vi "Mark Points Holder.vi"(2 "Actions":T1=enum."Read", 7 "(X, Y) Points":dbl[](array[numeric]), 13 "Zero Position (x, y)":dbl[](array[numeric])) -> (4 "Marked Points":cluster{dbl[], dbl[]}, 10 "X Zero (µm)":dbl, 15 "Y Zero (µm)":dbl)   [LabVIEW 2016]
uses:
  XY Sample Stage Controls/History Actions.ctl
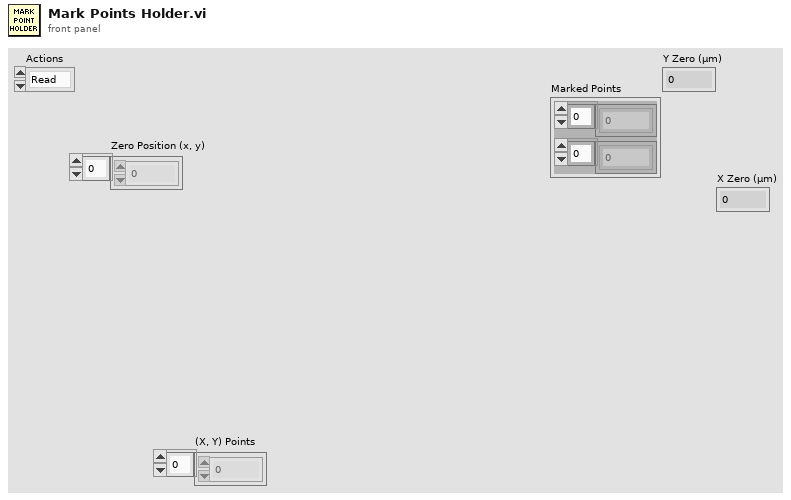
[diagram p1: front panel]
types:
  T1 = typedef "History Actions.ctl" = enum16{"Reset", "Write", "Read", "Set Zero"}
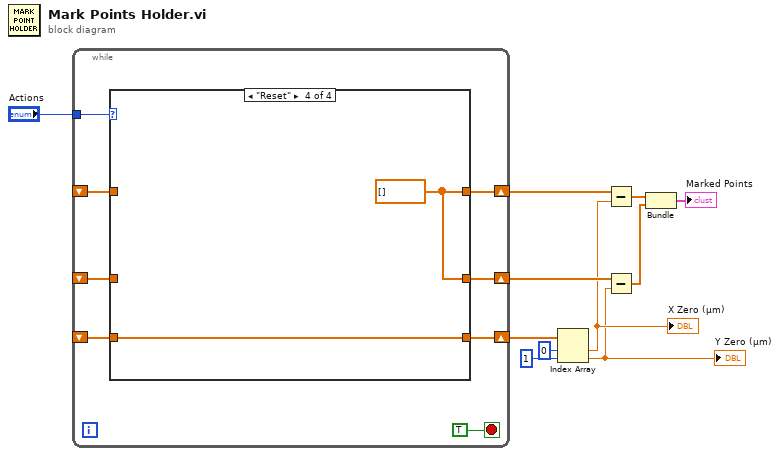
[diagram p0: block diagram]
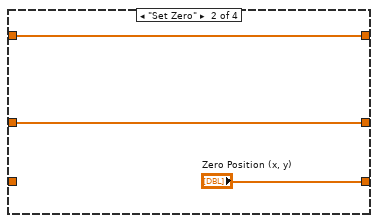
[diagram p3: hidden frame]
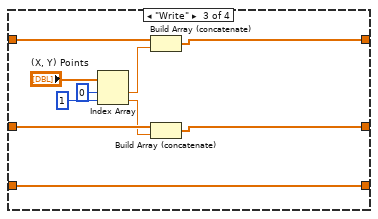
[diagram p4: hidden frame]
diagram:
  n1 = while {
    shift-right: [w17] -> w6
    shift-left: _ -> [w15]
    shift-right: [w16] -> w5
    shift-left: _ -> [w14]
    tunnel: "Actions" -> [w18]
    shift-right: [w13] -> w9
    shift-left: _ -> [w12]
    stop <- TRUE stop-if-true
    n2 = case shown="\"Reset\"" w18 {
      tunnel: [w22 w25 w28 w37] -> w17
      tunnel: [w21 w24 w27 w37] -> w16
      tunnel: w15 -> [w22 w25 w35 _]
      tunnel: w14 -> [w21 w24 w34 _]
      tunnel: [w20 "Zero Position (x, y)" w26 w36] -> w13
      tunnel: w12 -> [w20 _ w26 w36]
      frame "Read", Default {
      }
      frame "Set Zero" {
      }
      frame "Write" {
        n3 = Index Array(array="(X, Y) Points", index #1=0 ("index"), index #2=1 ("index")) -> (element #1=w30:dbl, element #2=w29:dbl)
        n4 = Build Array (concatenate)(w35, w30) -> (w28:dbl[])
        n5 = Build Array (concatenate)(w34, w29) -> (w27:dbl[])
      }
      frame "Reset" {
        w37 = dbl[] []
      }
    }
  }
  n6 = Index Array(array=w9, index #1=0 ("index"), index #2=1 ("index")) -> (element #1=w4:dbl, element #2=w3:dbl)
  "Y Zero (µm)" <- w3
  "X Zero (µm)" <- w4
  n7 = Subtract(x=w6, y=w4) -> (x-y=w2:dbl[])
  n8 = Subtract(x=w5, y=w3) -> (x-y=w1:dbl[])
  n9 = Bundle(w2, w1) -> (→"Marked Points":cluster{dbl[], dbl[]})  [unwired: 1 in]
